vi "Create Evaluations.vi"(8 "error in (no error)":errorcluster, 11 "IEvaluation in":refnum<class "NF Eval.lvclass">) -> (0 "error out":errorcluster, 2 "Evaluations Out":T1[](array[typedef]) {"Low Limit" format="%#_13g"; "SI Scaling" items=["femto"=-15, "pico"=-12, "nano"=-9, "micro"=-6, "milli"=-3, "percent"=-2, ""=0, "kilo"=3, "mega"=6, "giga"=9, "tera"=12]}, 3 "IEvaluation out":refnum<class "NF Eval.lvclass">)   [LabVIEW 2016, in "SeqAuto Evaluations.lvlib" / "NF Eval.lvclass"]
uses:
  NF Eval.lvclass
  C:/Sequence Automation/Plugins/SeqAuto IEvaluation.lvlibp/SeqAuto IEvaluation.lvclass
  Plugins/TestStand API Tools (TSAT).lvlibp/Evaluation Actions/Includes/Controls/TSAT Evaluation.ctl
  Plugins/TestStand API Tools (TSAT).lvlibp/Evaluation Actions/Includes/Controls/TSAT Eval SI Unit Scaling.ctl
  Plugins/TestStand API Tools (TSAT).lvlibp/Evaluation Actions/Includes/Controls/TSAT Evaluation Type.ctl
  NF Eval.lvclass/NF Eval.ctl
  Plugins/SeqAuto IEvaluation.lvlibp/Read Measurement Name.vi
  Plugins/TestStand API Tools (TSAT).lvlibp/Evaluation Actions/TSAT Evaluation Actions.lvlib
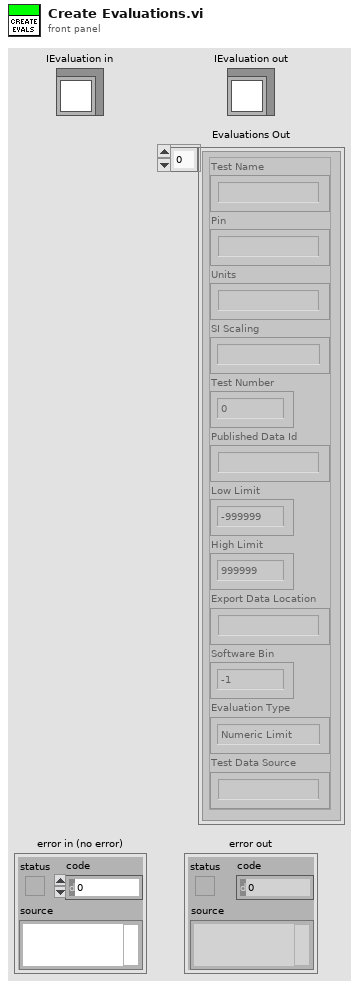
[diagram p1: front panel]
types:
  T1 = typedef "TestStand API Tools (TSAT).lvlibp/TSAT Evaluation Actions.lvlib/TSAT Evaluation.ctl" = cluster{"Test Name":string, "Pin":string, "Units":string, "SI Scaling":T2, "Test Number":i32, "Published Data Id":string, "Low Limit":dbl, "High Limit":dbl, "Export Data Location":string, "Software Bin":i64, "Evaluation Type":T3, "Test Data Source":string}
  T2 = typedef "TestStand API Tools (TSAT).lvlibp/TSAT Evaluation Actions.lvlib/TSAT Eval SI Unit Scaling.ctl" = i16
  T3 = typedef "TestStand API Tools (TSAT).lvlibp/TSAT Evaluation Actions.lvlib/TSAT Evaluation Type.ctl" = enum16{"Numeric Limit", "Pass/Fail", "None"}
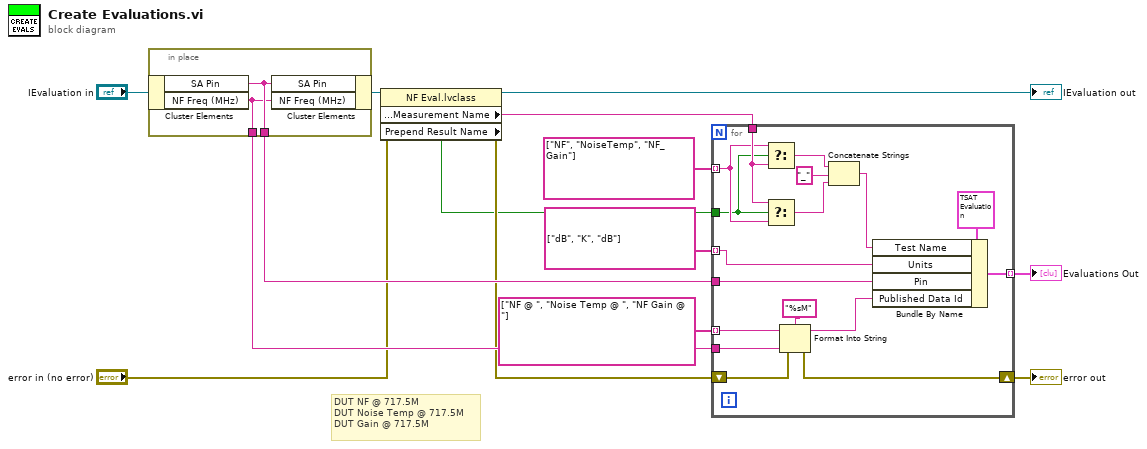
[diagram p0: block diagram]
diagram:
  # "DUT NF @ 717.5M\nDUT Noise Temp @ 717.5M\nDUT Gain @ 717.5M"
  n1 = in-place {
    in-place-border: [w16] -> w10
    in-place-border: [w15] -> w9
    n2 = in-place-cluster #1("IEvaluation in") -> ("SA Pin"=w16:string, "NF Freq (MHz)"=w15:string)
    n3 = in-place-cluster #1("SA Pin"=w16, "NF Freq (MHz)"=w15) -> (w13:refnum<class "NF Eval.lvclass">)
  }
  n4 = property class="NF Eval.lvclass"(reference=w13, error in="error in (no error)") -> (reference out=→"IEvaluation out":refnum<class "NF Eval.lvclass">, error out=w7:errorcluster, "Protected Methods:Measurement Name"=w11:string, "Prepend Result Name"=w1:bool)
  n5 = for {
    tunnel: w11 -> [w23]
    tunnel: w10 -> [w32]
    tunnel: w9 -> [w31]
    tunnel: [w26] -> w5 mode=indexing
    shift-right: [w27] -> w6
    shift-left: w7 -> [w28]
    tunnel: string[] ["NF @ ", "Noise Temp @ ", "NF Gain @ "] -> [w25] mode=indexing
    tunnel: string[] ["dB", "K", "dB"] -> [w24] mode=indexing
    tunnel: string[] ["NF", "NoiseTemp", "NF_Gain"] -> [w19] mode=indexing
    tunnel: w1 -> [w18]
    n6 = Select(t=w19, s=w18, f=w23) -> (s? t:f=w21:string)
    n7 = Select(t=w23, s=w18, f=w19) -> (s? t:f=w22:string)
    n8 = Format Into String(format string="%sM", initial string=w25, error in=w28, w31) -> (resulting string=w30:string, error out=w27:errorcluster)
    n9 = Concatenate Strings(w21, "_" ("string"), w22) -> (w17:string)
    n10 = Bundle By Name(cluster=T1 {"Test Name"="", "Pin"="", "Units"="dBm", "SI Scaling"=0, "Test Number"=0, "Published Data Id"="", "Low Limit"=-999999.0, "High Limit"=999999.0, "Export Data Location"="", "Software Bin"=-1, "Evaluation Type"=enum."Numeric Limit", "Test Data Source"=""} ("Evaluation"), "Test Name"=w17, "Units"=w24, "Pin"=w32, "Published Data Id"=w30) -> (w26:T1)
  }
  "error out" <- w6
  "Evaluations Out" <- w5
